vi "Close.vi"(8 "error in (no error)":errorcluster, 11 "Monkey in":refnum<class "Monkey.lvclass">) -> (0 "error out":errorcluster, 3 "Monkey out":refnum<class "Monkey.lvclass">)   [LabVIEW 2020, in "Monkey.lvlib" / "Monkey.lvclass"]
uses:
  Monkey.lvclass
  C:/Users/marco/Documents/GitHub_Lab/TALOS/talos/Ancestor/Ancestor/Ancestor.lvclass
  C:/Users/marco/Documents/GitHub_Lab/TALOS/talos/Father of all uServices/Father of all uServices/Father of all uServices.lvclass
  Ancestor/Ancestor/Ancestor.lvclass/Ancestor.ctl
  Guardian/Guardian Messages/Message to uService Msg/Message to uService Msg.lvclass/Message to uService Msg.ctl
  Ancestor/Ancestor/Read ID.vi
  Guardian/Guardian Messages/Message to uService Msg/Send Message to uService.vi
  Support VIs/Substitute Error.vi
  Support VIs/Generate Error.vi
  FGV/Error Memory/Get Error Description.vi
  Support VIs/Get PC name.vi
  Support VIs/Get Class Name.vi
  <vilib>/Utility/error.llb/Clear Errors.vi
  FGV/Error Memory/Error Memory Core.vi
  <vilib>/AdvancedString/Delimited String to 1D String Array.vi
  Support VIs/Circus Root Path.vi
  FGV/Error Memory/Error Crt Lvl checker.vi
  FGV/Error Memory/Error Memory Core.vi/40c8088d-b597-4017-91af-faa98e00292e.vi
  FGV/Error Memory/Error Memory Core.vi/d4a3ab98-063c-4e44-b43d-fbdcfe6c2be2.vi
  Father of all uServices/Father of all uServices/Father of all uServices.lvclass
  C:/Users/marco/Documents/GitHub_Lab/TALOS/builds/Actor Framework PPL/Actor Framework.lvlibp/1abvi3w/vi.lib/ActorFramework/Actor/Actor.lvclass
  Support VIs/Global Constants.vi
  builds/Actor Framework PPL/Actor Framework.lvlibp/1abvi3w/vi.lib/ActorFramework/Actor/Read Caller Enqueuer.vi
  builds/Actor Framework PPL/Actor Framework.lvlibp/1abvi3w/vi.lib/ActorFramework/Message Enqueuer/Enqueue.vi
  Support VIs/Global Memory.vi
  <vilib>/Utility/LVClass/Get LV Class Name.vi
  Support VIs/Is in Packed Library.vi
  Support VIs/TALOS Root path.vi
  Support VIs/Read CSV worksheet.vi
  <vilib>/Utility/error.llb/General Error Handler.vi
  Support VIs/Error Log.vi
  Guardian/Guardian Messages/Message to uService Msg/Message to uService Msg.lvclass
  Ancestor/Ancestor/Ancestor.lvclass
  <vilib>/Comparison/Equal/Equal Functor/Equal Functor.lvclass
  TALOS.lvlib
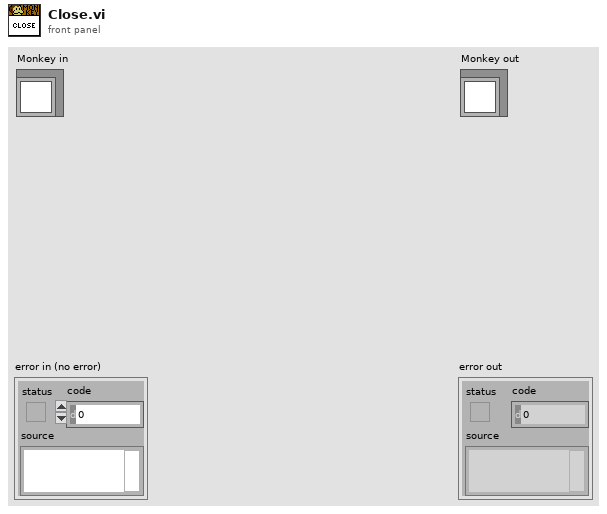
[diagram p1: front panel]
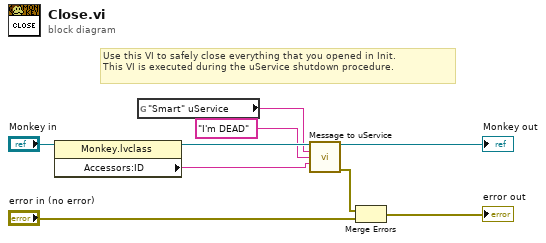
[diagram p0: block diagram]
diagram:
  # "Use this VI to safely close everything that you opened in Init.\nThis VI is executed during the uService shutdown procedure."
  n1 = property class="Monkey.lvclass"(reference="Monkey in") -> (reference out=w8:refnum<class "Monkey.lvclass">, "Accessors:ID"=w6:string)  [unwired: 1 in, 1 out]
  n2 = global read "Global Constants.vi" "\"Smart\" uService"() -> (w1:string)
  n3 = call "Message to uService.vi"("Father of all uServices in"=w8, "uService ID"=w1, "Message"="I'm DEAD", "Data"=w6) -> ("Father of all uServices out"=→"Monkey out":refnum<class "Monkey.lvclass">, "error out"=w3:errorcluster)  [unwired: 10 in]
  n4 = Merge Errors(w3, "error in (no error)") -> (→"error out":errorcluster)
